vi "SPI_CY_host.vi"() -> ()   [LabVIEW 2018]
uses:
  <vilib>/userdefined/High Color/nirio_resource_hc.ctl
  <vilib>/FPGAPlugInAG/PXI-7951R/niLvFpga_Open_PXI-7951R.vi
  <vilib>/FPGAPlugInAG/PXI-7951R/niLvFpga_Reset_PXI-7951R.vi
  <vilib>/FPGAPlugInAG/PXI-7951R/niLvFpga_Run_PXI-7951R.vi
  <vilib>/Utility/error.llb/Error Cluster From Error Code.vi
  <vilib>/rvi/errors/niLvFpgaAdjustHostInterfaceError.vi
  <vilib>/FPGAPlugInAG/PXI-7951R/niLvFpga_Close_PXI-7951R.vi
  <vilib>/rvi/interface/nirviOpenFPGA/nirviOpenFPGA.xnode
  FPGA Bitfiles/SPICY_FPGATarget_SPICYtarget_ZcIeO-4C02g.lvbitx
  <vilib>/rvi/interface/nirviMethod/nirviMethod.xnode
  <vilib>/rvi/interface/nirviReadWriteControl/nirviReadWriteControl.xnode
  <vilib>/rvi/interface/nirviCloseFPGA/nirviCloseFPGA.xnode
  <vilib>/rvi/errors/niLvFpgaMergeErrorWithErrorCode.vi
  NiFpgaLv.dll
  <vilib>/FPGAPlugInAG/PXI-7951R/niLvFpga_ReadFifo_PXI-7951R.vi
  <vilib>/FPGAPlugInAG/PXI-7951R/niLvFpga_WriteFifo_PXI-7951R.vi
panel:
  in  "Operation loop?":bool
  out "Status":bool=TRUE
  out "Address Error":i32[](array[numeric])
  out "TotalErrorAddress":i32
  out "TotalErrorBitsAddr":i32[](array[numeric])
  out "TotalErrorBits":i32
  out "Address Read":u32(slide)=2097152 scale=0.0..2097152.0
  out "WriteError?":bool
  out "WriteChipComplete":bool=TRUE
  out "Elements Remaining (Read)":u32
  out "Read":u8[](array[numeric]) format="%b"
  out "ReadChipComplete":bool=TRUE
  in  "Start Part":i32
  in  "ReadWords":u32=65536
  in  "ReadDelay":u8=1
  out "Write":u8[](array[numeric]) format="%b"
  out "size(s)":i32=65536
  out "Empty Elements Remaining (Write)":u32=65546
  in  "Parts":i32=32
  in  "Code":T1(ring)
  out "Address Write":u32(slide)=2097152 scale=0.0..2097152.0
  in  "Operation":enum16{"Read", "Write"}(ring)
  in  "Operation?":bool
  in  "Stop Test":bool
  in  "FPGA Resourse":T2="RIO0"
  in  "Current limit CH1":dbl=0.7 caption="Current limit CH0" format="%#_13g"
  in  "Voltage CH1, V":dbl=3.3 caption="Voltage level CH0" format="%#_13g"
  out "Voltage CH1, V":dbl=0.0005629324288814687
  out "Current CH1,A":dbl=-7.272896300718331e-07
  out "Current":dbl(knob)=8.655859624107152e-05 scale=0.0..0.7
  out "Voltage CH0, V":dbl=0.00020438404052728563
  out "Current CH0,A":dbl=8.655859624107152e-05
  in  "Voltage CH0, V":dbl=3.3 caption="Voltage level CH0" format="%#_13g"
  in  "Power Enable":bool caption="Output enabled CH0"
  in  "Current limit CH0":dbl=0.7 format="%#_13g"
  in  "Power Resource":refnum<k15>="PXI1Slot3"
  # "Error Statistics"
  # "32 max"
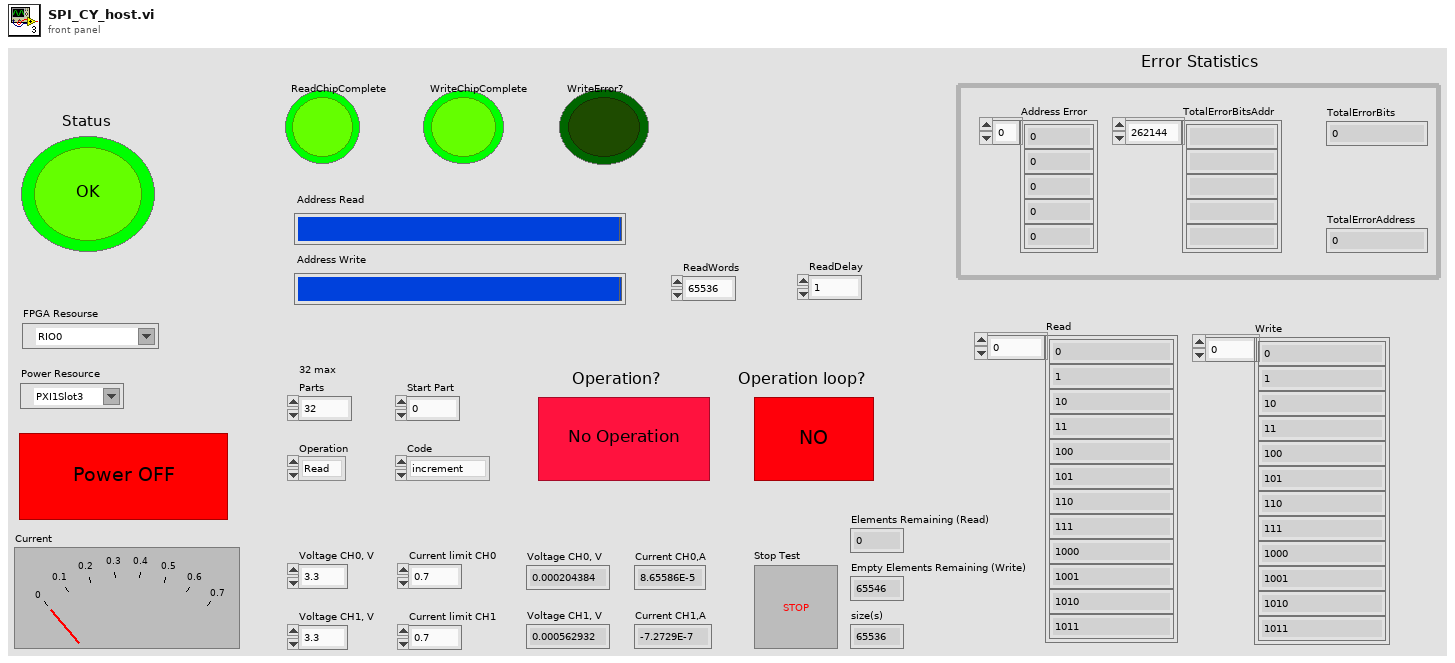
[diagram p1: front panel]
types:
  T1 = enum16{"increment", "decrement", "random", "Chess", "NChess", "One", "Zero"}
  T2 = typedef "nirio_resource_hc.ctl" = tag
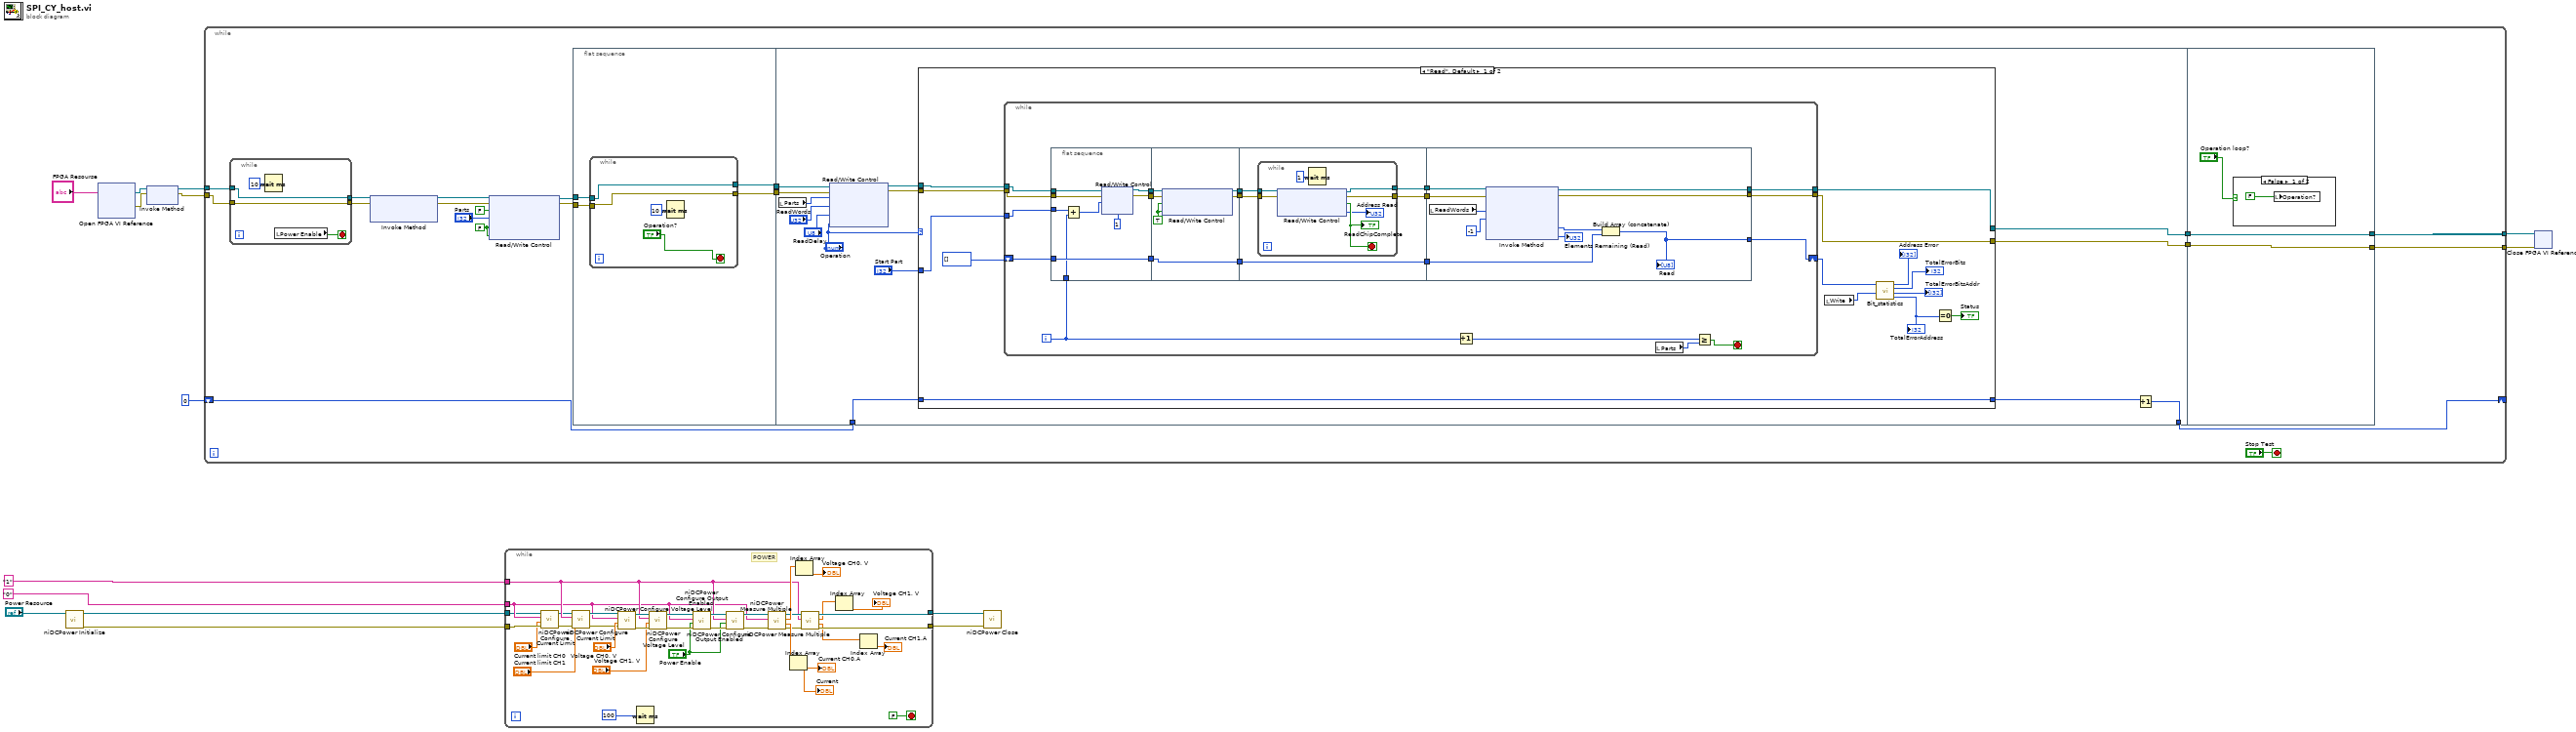
[diagram p0: block diagram]
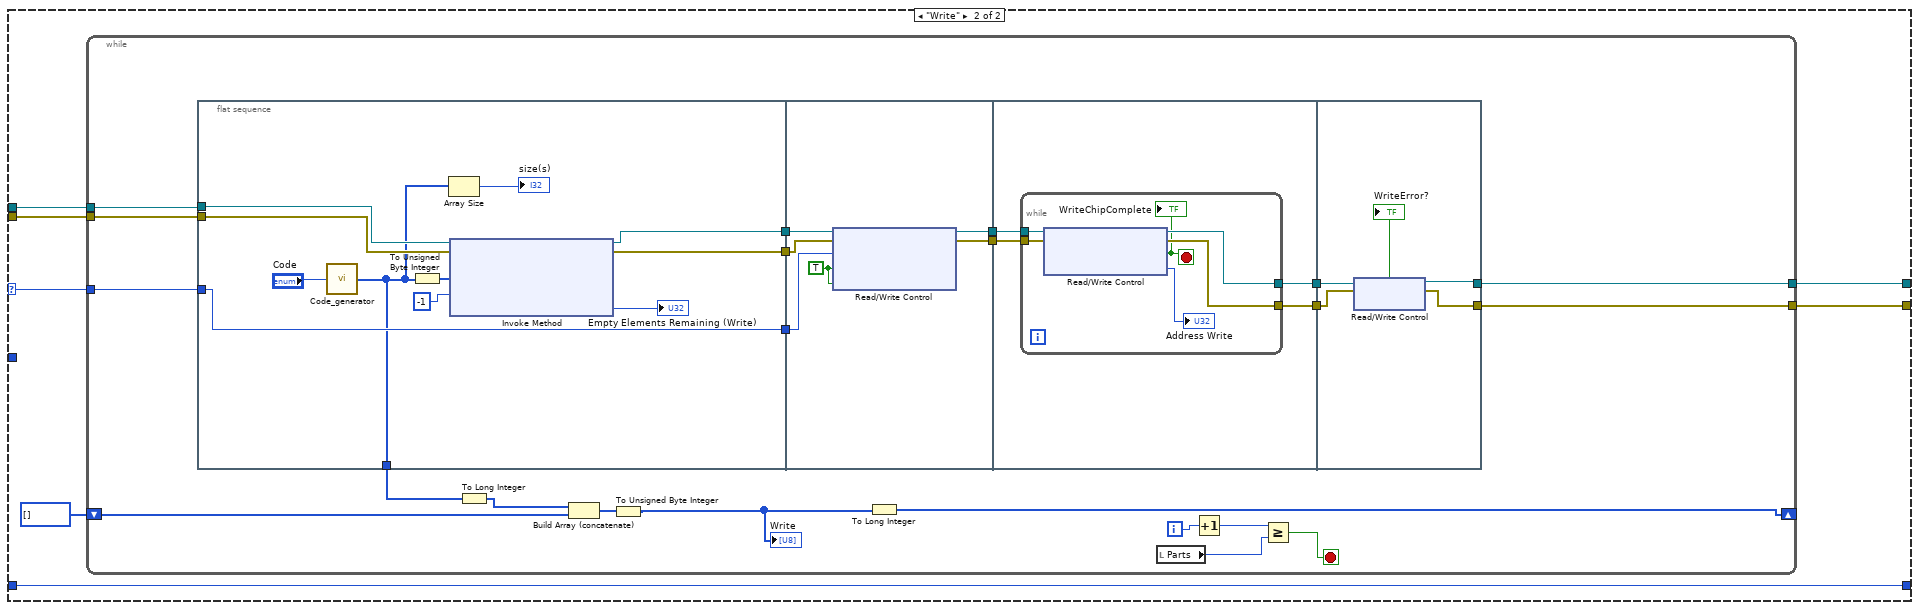
[diagram p2: hidden frame]
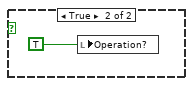
[diagram p3: hidden frame]
diagram:
  n1 = call <instrlib>:"niDCPower Initialize.vi"("resource name"="Power Resource") -> ("error out"=w10:errorcluster, "instrument handle out"=w9:refnum<k15>)  [unwired: 3 in, 6 out]
  n2 = xnode "Open FPGA VI Reference"("resource name"="FPGA Resourse") -> ("FPGA VI Reference Out"=w6:refnum<k20>, "error out"=w7:errorcluster)  [unwired: 1 in]
  n3 = xnode "Invoke Method"("FPGA VI Reference In"=w6, "error in"=w7) -> ("FPGA VI Reference Out"=w2:refnum<k20>, "error out"=w1:errorcluster)
  n4 = while {
    shift-right: [w29] -> _
    shift-left: 0 -> [w30]
    tunnel: [w17] -> w4
    tunnel: [w16] -> w3
    tunnel: w2 -> [w19]
    tunnel: w1 -> [w18]
    stop <- "Stop Test" stop-if-true
    w24 = FALSE ("NextPart")
    n5 = while {
      tunnel: [w37] -> w26
      tunnel: [w36] -> w27
      tunnel: w19 -> [w37]
      tunnel: w18 -> [w36]
      stop <- w39 stop-if-true
      n6 = Wait (ms)(milliseconds to wait=u32 10) -> ()  [unwired: 1 out]
      n7 = local read "Power Enable"() -> (w39:bool)
    }
    n8 = xnode "Invoke Method"("FPGA VI Reference In"=w26, "error in"=w27) -> ("FPGA VI Reference Out"=w23:refnum<k20>, "error out"=w22:errorcluster)  [unwired: 1 in]
    n9 = xnode "Read/Write Control"("FPGA VI Reference In"=w23, "error in"=w22, "Stop"=FALSE, "Parts"="Parts", "NextPart"=w24, "OperationComplete"=w24) -> ("FPGA VI Reference Out"=w21:refnum<k20>, "error out"=w20:errorcluster)
    n10 = flat-sequence {
      tunnel: w21 -> [w43]
      tunnel: w20 -> [w42]
      tunnel: [w41] -> w32
      tunnel: [w40] -> w31
      tunnel: [w61] -> w34
      tunnel: [w60] -> w33
      tunnel: w32 -> [w57]
      tunnel: w31 -> [w56]
      tunnel: w30 -> [w51]
      tunnel: [w49] -> w29
      tunnel: w34 -> [w195]
      tunnel: w33 -> [w196]
      tunnel: [w196] -> w17
      tunnel: [w195] -> w16
      frame #0 {
        n11 = while {
          tunnel: w43 -> [w46]
          tunnel: w42 -> [w45]
          tunnel: [w46] -> w41
          tunnel: [w45] -> w40
          stop <- "Operation?" stop-if-true
          n12 = Wait (ms)(milliseconds to wait=u32 10) -> ()  [unwired: 1 out]
        }
      }
      frame #1 {
        n13 = local read "Parts"() -> (w52:i32)
        n14 = xnode "Read/Write Control"("FPGA VI Reference In"=w57, "error in"=w56, "Parts"=w52, "ReadWords"="ReadWords", "ReadDelay"="ReadDelay", "SelectOperation"="Operation") -> ("FPGA VI Reference Out"=w59:refnum<k20>, "error out"=w58:errorcluster)
        n15 = case shown="\"Read\", Default" "Operation" {
          selector: "Operation" -> [_ w135]
          tunnel: [w71 w139] -> w61
          tunnel: [w72 w133] -> w60
          tunnel: w59 -> [w75 w138]
          tunnel: w58 -> [w74 w137]
          tunnel: w51 -> [w69 w134]
          tunnel: [w69 w134] -> w50
          tunnel: "Start Part" -> [w70 _]
          frame "Read", Default {
            n16 = while {
              tunnel: w75 -> [w95]
              tunnel: w74 -> [w94]
              shift-right: [w83] -> w68
              shift-left: u8[] [] -> [w87]
              tunnel: [w82] -> w72
              tunnel: [w81] -> w71
              tunnel: w70 -> [w77]
              i -> [w76]
              stop <- w80 stop-if-true
              n17 = flat-sequence {
                tunnel: w95 -> [w104]
                tunnel: w94 -> [w103]
                tunnel: [w102] -> w93
                tunnel: [w101] -> w92
                tunnel: w87 -> [w100]
                tunnel: [w100] -> w86
                tunnel: w77 -> [w98]
                tunnel: w76 -> [w97]
                tunnel: w93 -> [w110]
                tunnel: w92 -> [w109]
                tunnel: [w107] -> w91
                tunnel: [w106] -> w90
                tunnel: w86 -> [w105]
                tunnel: [w105] -> w84
                tunnel: w91 -> [w115]
                tunnel: w90 -> [w114]
                tunnel: [w113] -> w89
                tunnel: [w112] -> w88
                tunnel: [w111] -> w85
                tunnel: w84 -> [w111]
                tunnel: w89 -> [w132]
                tunnel: w88 -> [w131]
                tunnel: w85 -> [w129]
                tunnel: [w123] -> w83
                tunnel: [w124] -> w82
                tunnel: [w125] -> w81
                frame #0 {
                  n18 = Add(x=w98, y=w97) -> (x+y=w96:i32)
                  n19 = xnode ("Read/Write Control")("FPGA VI Reference In"=w104, "error in"=w103, "i"=w96, "Parts"=1) -> ("FPGA VI Reference Out"=w102:refnum<k20>, "error out"=w101:errorcluster)
                }
                frame #1 {
                  w108 = TRUE ("NextPart")
                  n20 = xnode ("Read/Write Control")("FPGA VI Reference In"=w110, "error in"=w109, "OperationComplete"=w108, "NextPart"=w108) -> ("FPGA VI Reference Out"=w107:refnum<k20>, "error out"=w106:errorcluster)
                }
                frame #2 {
                  n21 = while {
                    tunnel: w115 -> [w122]
                    tunnel: w114 -> [w121]
                    tunnel: [w118] -> w113
                    tunnel: [w117] -> w112
                    stop <- w119 stop-if-true
                    n22 = xnode ("Read/Write Control")("FPGA VI Reference In"=w122, "error in"=w121) -> ("FPGA VI Reference Out"=w118:refnum<k20>, "error out"=w117:errorcluster, "ReadChipComplete"=w119:bool, "Addr Read"=→"Address Read":u32)
                    "ReadChipComplete" <- w119
                    n23 = Wait (ms)(milliseconds to wait=u32 1) -> ()  [unwired: 1 out]
                  }
                }
                frame #3 {
                  n24 = local read "ReadWords"() -> (w126:u32)
                  n25 = xnode "Invoke Method"("FPGA VI Reference In"=w132, "error in"=w131, "Number of Elements"=w126, "Timeout (ms)"=-1) -> ("FPGA VI Reference Out"=w124:refnum<k20>, "error out"=w125:errorcluster, "Data"=w128:u8[], "Elements Remaining"=→"Elements Remaining (Read)":u32)
                  n26 = Build Array (concatenate)(w128, w129) -> (w123:u8[])
                  "Read" <- w123
                }
              }
              n27 = Increment(x=w76) -> (x+1=w78:i32)
              n28 = local read "Parts"() -> (w79:i32)
              n29 = Greater Or Equal?(x=w78, y=w79) -> (x >= y?=w80:bool)
            }
            n30 = local read "Write"() -> (w67:u8[])
            n31 = call "Bit_statistics.vi"("Write Code"=w67, "Read Code"=w68) -> ("TotalErrorAddress"=w63:i32, "TotalErrorBitsAddr"=→"TotalErrorBitsAddr":i32[], "TotalErrorBits"=→"TotalErrorBits":i32, "Address Error"=→"Address Error":i32[])  [unwired: 2 in]
            "TotalErrorAddress" <- w63
            n32 = Equal To 0?(x=w63) -> (x = 0?=→"Status":bool)
          }
          frame "Write" {
            n33 = while {
              tunnel: [w140] -> w139
              tunnel: [w141] -> w133
              tunnel: w138 -> [w158]
              tunnel: w137 -> [w157]
              shift-right: [w142] -> _
              shift-left: i32[] [] -> [w150]
              tunnel: w135 -> [w152]
              i -> [w161]
              stop <- w159 stop-if-true
              n34 = flat-sequence {
                tunnel: w158 -> [w172]
                tunnel: w157 -> [w171]
                tunnel: [w170] -> w156
                tunnel: [w169] -> w155
                tunnel: w152 -> [w164]
                tunnel: [w164] -> w151
                tunnel: [w162] -> w144
                tunnel: w156 -> [w178]
                tunnel: w155 -> [w177]
                tunnel: [w176] -> w154
                tunnel: [w175] -> w153
                tunnel: w151 -> [w174]
                tunnel: w154 -> [w182]
                tunnel: w153 -> [w181]
                tunnel: [w180] -> w148
                tunnel: [w179] -> w147
                tunnel: w148 -> [w193]
                tunnel: w147 -> [w192]
                tunnel: [w190] -> w141
                tunnel: [w189] -> w140
                frame #0 {
                  n35 = call "Code_generator.vi"("Code"="Code") -> ("Array"=w162:u16[])
                  n36 = To Unsigned Byte Integer(number=w162) -> (unsigned 8bit integer=w163:u8[])
                  n37 = Array Size(array=w162) -> (size(s)=→"size(s)":i32)
                  n38 = xnode "Invoke Method"("FPGA VI Reference In"=w172, "error in"=w171, "Data"=w163, "Timeout (ms)"=-1) -> ("FPGA VI Reference Out"=w170:refnum<k20>, "error out"=w169:errorcluster, "Empty Elements Remaining"=→"Empty Elements Remaining (Write)":u32)
                }
                frame #1 {
                  w173 = TRUE ("OperationComplete")
                  n39 = xnode ("Read/Write Control")("FPGA VI Reference In"=w178, "error in"=w177, "SelectOperation"=w174, "OperationComplete"=w173, "NextPart"=w173) -> ("FPGA VI Reference Out"=w176:refnum<k20>, "error out"=w175:errorcluster)
                }
                frame #2 {
                  n40 = while {
                    tunnel: w182 -> [w188]
                    tunnel: w181 -> [w187]
                    tunnel: [w186] -> w180
                    tunnel: [w185] -> w179
                    stop <- w183 stop-if-true
                    n41 = xnode ("Read/Write Control")("FPGA VI Reference In"=w188, "error in"=w187) -> ("FPGA VI Reference Out"=w186:refnum<k20>, "error out"=w185:errorcluster, "WriteChipComplete"=w183:bool, "Addr"=→"Address Write":u32)
                    "WriteChipComplete" <- w183
                  }
                }
                frame #3 {
                  n42 = xnode "Read/Write Control"("FPGA VI Reference In"=w193, "error in"=w192) -> ("FPGA VI Reference Out"=w190:refnum<k20>, "error out"=w189:errorcluster, "WriteError"=→"WriteError?":bool)
                }
              }
              n43 = To Long Integer(number=w144) -> (32bit integer=w145:i32[])
              n44 = Build Array (concatenate) "Build Array"(w145, w150) -> (w146:i32[])
              n45 = To Unsigned Byte Integer(number=w146) -> (unsigned 8bit integer=w143:u8[])
              "Write" <- w143
              n46 = To Long Integer(number=w143) -> (32bit integer=w142:i32[])
              n47 = local read "Parts"() -> (w149:i32)
              n48 = Increment(x=w161) -> (x+1=w160:i32)
              n49 = Greater Or Equal?(x=w160, y=w149) -> (x >= y?=w159:bool)
            }
          }
        }
        n50 = Increment(x=w50) -> (x+1=w49:i32)
      }
      frame #2 {
        n51 = case shown="False" "Operation loop?" {
          frame False {
            n52 = local write "Operation?"(FALSE ("Operation Complete")) -> ()
          }
          frame True {
            n53 = local write "Operation?"(TRUE ("Operation Complete")) -> ()
          }
        }
      }
    }
  }
  n54 = while {
    tunnel: "0" ("Channel name") -> [w204]
    tunnel: [w216] -> w14
    tunnel: [w217] -> w13
    tunnel: "1" ("Channel name") -> [w208]
    tunnel: w10 -> [w205]
    tunnel: w9 -> [w203]
    stop <- FALSE stop-if-true
    # "POWER"
    n55 = call <instrlib>:"niDCPower Configure Current Limit.vi"("error in (no error)"=w205, "current limit"="Current limit CH0", "channel name"=w204, "instrument handle"=w203) -> ("error out"=w202:errorcluster, "instrument handle out"=w201:refnum<k15>)  [unwired: 6 in]
    n56 = call <instrlib>:"niDCPower Configure Current Limit.vi"("error in (no error)"=w202, "current limit"="Current limit CH1", "channel name"=w208, "instrument handle"=w201) -> ("error out"=w207:errorcluster, "instrument handle out"=w206:refnum<k15>)  [unwired: 6 in]
    n57 = call <instrlib>:"niDCPower Configure Voltage Level.vi"("error in (no error)"=w207, "voltage level"="Voltage CH0, V", "channel name"=w204, "instrument handle"=w206) -> ("error out"=w227:errorcluster, "instrument handle out"=w226:refnum<k15>)  [unwired: 6 in]
    n58 = Wait (ms)(milliseconds to wait=u32 100) -> ()  [unwired: 1 out]
    n59 = call <instrlib>:"niDCPower Configure Voltage Level.vi"("error in (no error)"=w227, "voltage level"="Voltage CH1, V", "channel name"=w208, "instrument handle"=w226) -> ("error out"=w220:errorcluster, "instrument handle out"=w221:refnum<k15>)  [unwired: 6 in]
    n60 = call <instrlib>:"niDCPower Configure Output Enabled.vi"("error in (no error)"=w220, "output enabled"="Power Enable", "channel name"=w204, "instrument handle"=w221) -> ("error out"=w225:errorcluster, "instrument handle out"=w224:refnum<k15>)  [unwired: 6 in]
    n61 = call <instrlib>:"niDCPower Configure Output Enabled.vi"("error in (no error)"=w225, "output enabled"="Power Enable", "channel name"=w208, "instrument handle"=w224) -> ("error out"=w222:errorcluster, "instrument handle out"=w223:refnum<k15>)  [unwired: 6 in]
    n62 = call <instrlib>:"niDCPower Measure Multiple.vi"("error in (no error)"=w222, "channel name"=w204, "instrument handle"=w223) -> ("error out"=w219:errorcluster, "current measurements"=w230:dbl[], "voltage measurements"=w231:dbl[], "instrument handle out"=w218:refnum<k15>)  [unwired: 5 in]
    n63 = Index Array(array=w230) -> (element=→"Current CH0,A" →"Current":dbl)  [unwired: 1 in]
    n64 = Index Array(array=w231) -> (element=→"Voltage CH0, V":dbl)  [unwired: 1 in]
    n65 = call <instrlib>:"niDCPower Measure Multiple.vi"("error in (no error)"=w219, "channel name"=w208, "instrument handle"=w218) -> ("error out"=w216:errorcluster, "current measurements"=w215:dbl[], "voltage measurements"=w211:dbl[], "instrument handle out"=w217:refnum<k15>)  [unwired: 5 in]
    n66 = Index Array(array=w211) -> (element=→"Voltage CH1, V":dbl)  [unwired: 1 in]
    n67 = Index Array(array=w215) -> (element=→"Current CH1,A":dbl)  [unwired: 1 in]
  }
  n68 = call <instrlib>:"niDCPower Close.vi"("error in (no error)"=w14, "instrument handle"=w13) -> ()  [unwired: 9 in, 1 out]
  n69 = xnode "Close FPGA VI Reference"("FPGA VI Reference In"=w4, "error in"=w3) -> ()  [unwired: 1 out]
